vi "Get Substring.vi"(8 "error in":errorcluster, 9 "offset and length":T1, 11 "string in":string) -> (0 "error out":errorcluster, 2 "substring":string)   [LabVIEW 2011]
uses:
  Type Defs/Node Info - Cluster.ctl
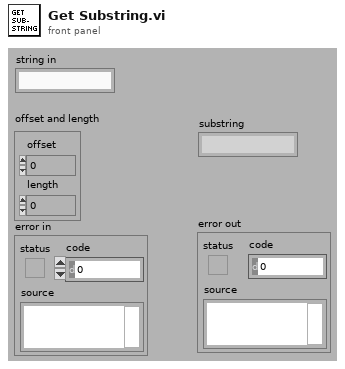
[diagram p1: front panel]
types:
  T1 = typedef "Node Info - Cluster.ctl" = cluster{"offset":i32, "length":i32}
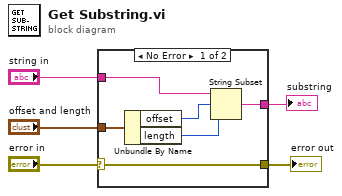
[diagram p0: block diagram]
diagram:
  n1 = case shown="No Error" "error in" {
    selector: "error in" -> [w6 w12]
    tunnel: "offset and length" -> [w11 _]
    tunnel: "string in" -> [w10 _]
    tunnel: [w7 _] -> w4
    tunnel: [w6 w12] -> w5
    frame No Error {
      n2 = Unbundle By Name(w11) -> ("offset"=w9:i32, "length"=w8:i32)
      n3 = String Subset(string=w10, offset (0)=w9, length (rest)=w8) -> (substring=w7:string)
    }
    frame Error {
    }
  }
  "error out" <- w5
  "substring" <- w4
